vi "UI SaveAs Config.vi"(8 "error in (no error)":errorcluster, 11 "UIActorTop in":refnum<class "UIActorTop.lvclass">) -> (0 "error out":errorcluster, 3 "UIActorTop out":refnum<class "UIActorTop.lvclass">)   [LabVIEW 2021, in "AbstractActorTemplate.lvlib" / "UIActorTop.lvclass"]
uses:
  <userlib>/John_Lib/AbstractActorTemplate/AbstractActorTemplate/UIActorTop.lvclass
  <vilib>/ActorFramework/Message Enqueuer/Message Enqueuer.lvclass/Message Enqueuer.ctl
  <vilib>/ActorFramework/Message Enqueuer/Enqueue.vi
  <userlib>/John_Lib/AbstractActorTemplate/UIActorTop Messages/UI SaveAs Config Msg/UI SaveAs Config Msg.lvclass
  C:/Program Files (x86)/National Instruments/LabVIEW 2021/vi.lib/ActorFramework/Message/Message.lvclass
  <vilib>/ActorFramework/Message Priority Queue/Priority Enqueue.vi
  <vilib>/ActorFramework/Message Enqueuer/Message Enqueuer.lvclass
  <userlib>/John_Lib/AbstractActorTemplate/AbstractActorTemplate/UIActorTop.lvclass/UIActorTop.ctl
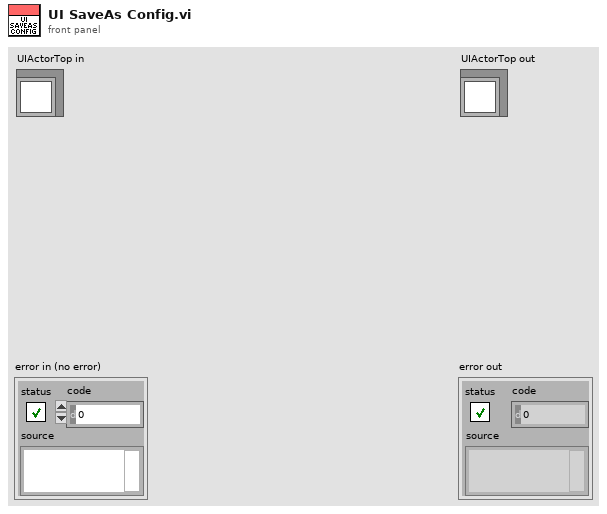
[diagram p1: front panel]
types:
  T1 = map{string, refnum<class "Message Enqueuer.lvclass">}
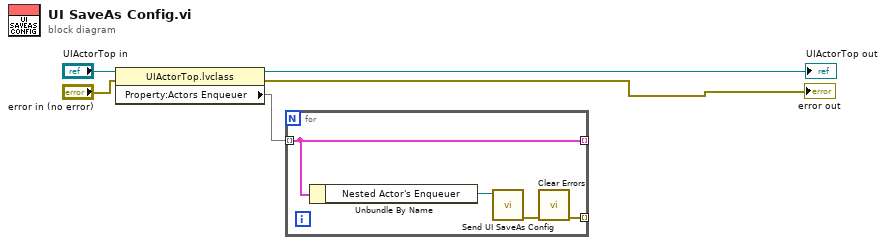
[diagram p0: block diagram]
diagram:
  n1 = property class="UIActorTop.lvclass"(reference="UIActorTop in", error in="error in (no error)") -> (reference out=→"UIActorTop out":refnum<class "UIActorTop.lvclass">, error out=→"error out":errorcluster, "Property:Actors Enqueuer"=w5:T1)
  n2 = for {
    tunnel: [w9] -> _ mode=indexing
    tunnel: w5 -> [w9] mode=indexing
    tunnel: [w8] -> _ mode=indexing
    n3 = Unbundle By Name(w9) -> ("Nested Actor's Enqueuer"=w7:refnum<class "Message Enqueuer.lvclass">)
    n4 = call <userlib>:"Send UI SaveAs Config.vi"("Message Enqueuer"=w7) -> ("error out"=w6:errorcluster)  [unwired: 9 in, 1 out]
    n5 = call <vilib>:"Clear Errors.vi"("error in (no error)"=w6) -> ("error out"=w8:errorcluster)  [unwired: 5 in, 1 out]
  }
